vi "Init Server.vi"(8 "error in (no error)":errorcluster, 11 "Timer Demo App in":refnum<class "Timer Demo App.lvclass">) -> (0 "error out":errorcluster, 3 "Timer Demo App out":refnum<class "Timer Demo App.lvclass">)   [LabVIEW 2020, in "Timer Demo.lvlib" / "Timer Demo App.lvclass"]
uses:
  Timer Demo App.lvclass
  Timer Demo App.lvclass/Timer Demo App.ctl
  HTTP Server/Server/Server.lvclass
  TimerStatusController/TimerStatusController.lvclass
  TimerActionController/TimerActionController.lvclass
  C:/dev/illuminated-g/lv-http-server/HTTP Server/Controller/Controller.lvclass
  C:/dev/illuminated-g/lv-http-server/HTTP Server/Handler/Handler.lvclass
  C:/dev/illuminated-g/lv-http-server/Test/Timer Demo/TimerStatusController/TimerStatusController.lvclass
  C:/dev/illuminated-g/lv-http-server/Test/Timer Demo/TimerActionController/TimerActionController.lvclass
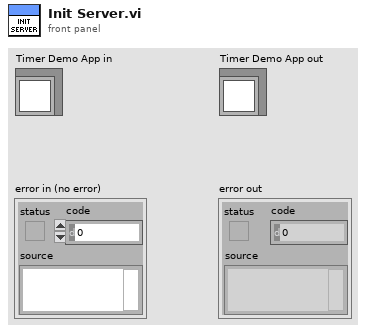
[diagram p1: front panel]
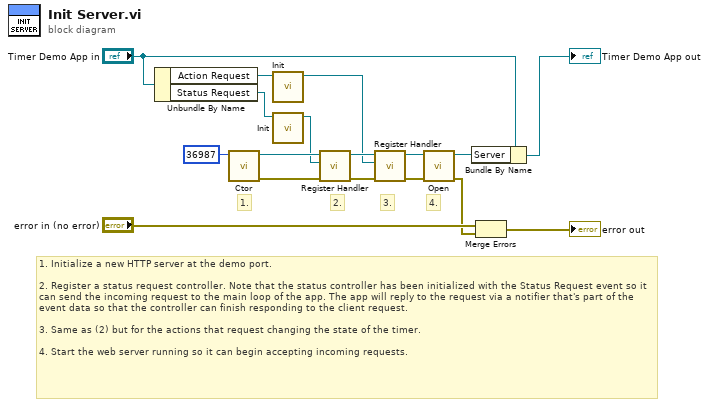
[diagram p0: block diagram]
diagram:
  # "1. Initialize a new HTTP server at the demo port.\n\n2. Register a status request controller. Note that the status controller has been initialized with the Status Request event so it can send the incoming request to the main loop of the app. The app will reply to the request via a notifier that's part of the event data so that the controller can finish responding to the client request.\n\n3. Same as (2) but for the actions that request changing the state of the timer.\n\n4. Start the web server running so it can begin accepting incoming requests."
  # "4."
  # "3."
  # "2."
  # "1."
  n1 = Unbundle By Name("Timer Demo App in") -> ("Action Request"=w10:refnum<user-event>, "Status Request"=w12:refnum<user-event>)
  n2 = call "Ctor.vi"("HTTP Port (80)"=u16 36987) -> ("error out"=w15:errorcluster, "Server out"=w16:refnum<class "Server.lvclass">)  [unwired: 9 in]
  n3 = call "Init.vi"("Action Request"=w10) -> ("TimerActionController out"=w7:refnum<class "TimerActionController.lvclass">)  [unwired: 9 in, 1 out]
  n4 = call "Init.vi"("Status Request"=w12) -> ("TimerStatusController out"=w11:refnum<class "TimerStatusController.lvclass">)  [unwired: 9 in, 1 out]
  n5 = call "Register Handler.vi"("error in (no error)"=w15, "Handler"=w11, "Server in"=w16) -> ("error out"=w8:errorcluster, "Server out"=w9:refnum<class "Server.lvclass">)  [unwired: 7 in]
  n6 = call "Register Handler.vi"("error in (no error)"=w8, "Handler"=w7, "Server in"=w9) -> ("error out"=w3:errorcluster, "Server out"=w4:refnum<class "Server.lvclass">)  [unwired: 7 in]
  n7 = call "Open.vi"("error in (no error)"=w3, "Server in"=w4) -> ("error out"=w1:errorcluster, "Server out"=w2:refnum<class "Server.lvclass">)  [unwired: 8 in]
  n8 = Bundle By Name(cluster="Timer Demo App in", "Server"=w2) -> (→"Timer Demo App out":refnum<class "Timer Demo App.lvclass">)
  n9 = Merge Errors("error in (no error)", w1) -> (→"error out":errorcluster)
